vi "Get Reply Data.vi"(8 "error in (no error)":errorcluster, 9 "Data Msg in":refnum<class "Data Msg.lvclass">, 10 "Actor in":refnum<class "Actor.lvclass">, 11 "Replay Message":refnum<class "ReplayData Msg.lvclass">) -> (0 "error out":errorcluster, 1 "Data Msg out":refnum<class "Data Msg.lvclass">, 2 "Actor out":refnum<class "Actor.lvclass">, 3 "Replay Message out":refnum<class "ReplayData Msg.lvclass">, 4 "error?":bool)   [LabVIEW 2014, in "ReplayData Msg.lvclass"]
doc: "(<B>Filename</B>: Actor Framework.lvlib:Message.lvclass:Do.vi)\n\nDefines what a message does when it is received by an actor. Generally, a message instructs an actor to invoke one of its methods. By default, this method does nothing. A child class must override it to define behavior. Create a child class by using the Actor Framework Message Maker dialog box."
uses:
  ReplayData Msg.lvclass
  <vilib>/ActorFramework/Actor/Actor.lvclass
  Data Msg/Data Msg.lvclass
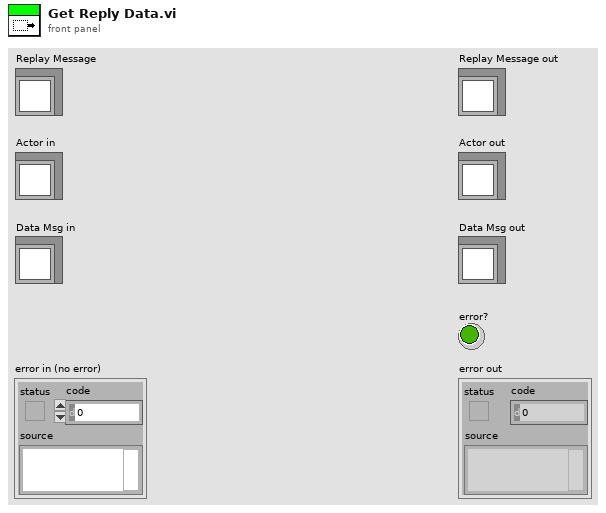
[diagram p1: front panel]
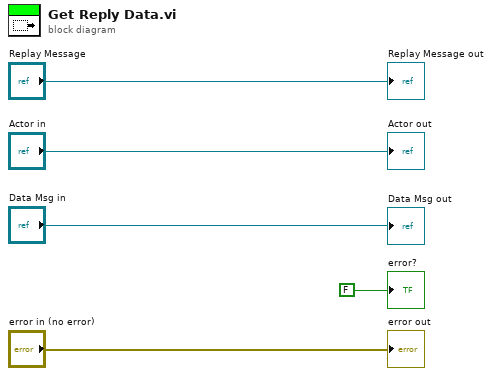
[diagram p0: block diagram]
diagram:
  "error out" <- "error in (no error)"
  "Actor out" <- "Actor in"
  "Replay Message out" <- "Replay Message"
  "Data Msg out" <- "Data Msg in"
  "error?" <- FALSE
